vi "Main Read Data From VeriStand.vi"(8 "error in":errorcluster, 10 "Outgoing Cyclic Configuraiton":T1 {"Outgoing Cyclic Frame"."Transmit Propreties"."Transmit Time" format="%#_p"}, 11 "internal data":T6={"J1939 XNET Settings"={"XNET Database"="", "XNET Cluster"="", "CAN port"="", "Baud rate [Bd]"=0, "J1939 Network Address"=0, "Name"=0, "Termination"=0}, "j1939 queues"={"Processed Outgoing"=refnum, "Process Outgoing"=refnum, "stop notifier"=refnum, "error queue"=refnum, "active dtc"=refnum, "processed inc"=refnum}, "fgv references"={"BAM Buffer"=refnum, "CM Buffer"=refnum, "CM Gen"=refnum, "BAM Gen"=refnum, "Address Claims"=refnum, "RQST"=refnum, "scaling lut"=refnum, "data lut"=refnum, "cyclic scheduler"=refnum}, "frame in"="", "frame out"="", "timing"={"tb to j1939 queue timeout"=100, "j1939 to tb queue timeout"=100, "dtc loop period (ms)"=100, "CAN in loop period (ms)"=100, "process incoming queue timeout (ms)"=100, "Outgoing Write Decimation"=0, "process outgoing loop rate (ms)"=0, "periodic outgoing queue timeout (ms)"=10, "CAN out queue timeout (ms)"=100}}) -> ()   [LabVIEW 2013, in "J1939.lvlib"]
uses:
  J1939.lvlib
  API Types/Internal Data.ctl
  API Types/XNET Settings.ctl
  API Types/Setup Information Cluster.ctl
  API Types/CAN Outgoing Message Cluster.ctl
  API Types/Convert DTCs Cluster.ctl
  <vilib>/xnet/xnet.llb/XNET Frame CAN.ctl
  <vilib>/xnet/xnet.llb/XNET Frame Type CAN.ctl
  TP/TP List References.ctl
  BAM/BAM Buffer Connections List_Ref.ctl
  Connection Mode/Connection Mode Generation Connection Ref.ctl
  BAM/BAM Generation Connections List_Ref.ctl
  LUTs/J1939 Address Table Reference.ctl
  RQST/RQST Lookup Table Reference.ctl
  LUTs/J1939 Conversion Lookup Table Reference.ctl
  LUTs/J1939 Data Lookup Table Reference.ctl
  LUTs/Cyclic Frame Scheduler Lut Reference.ctl
  Configuration/TypeDefs/timing configuration.ctl
  CD/CD Outgoing Cyclic Configuration.ctl
  CD/CD Outgoing Cyclic Frame Pairs.ctl
  API Types/XNET Frame Event Properties.ctl
  module/configuration/Signal Mapping.ctl
  <vilib>/NI/Tag Bus/tag/Data Type.ctl
  Conversion Lookup Table Get Conversion Parameter.vi
  <vilib>/xnet/xnet.llb/XNET Convert.vi
  <vilib>/xnet/xnet.llb/XNET Convert (Signal to Frame Raw).vi
  <vilib>/NI/Tag Bus/tag/tag descriptor.lvclass
  module/configuration/J1939 configuration.lvclass
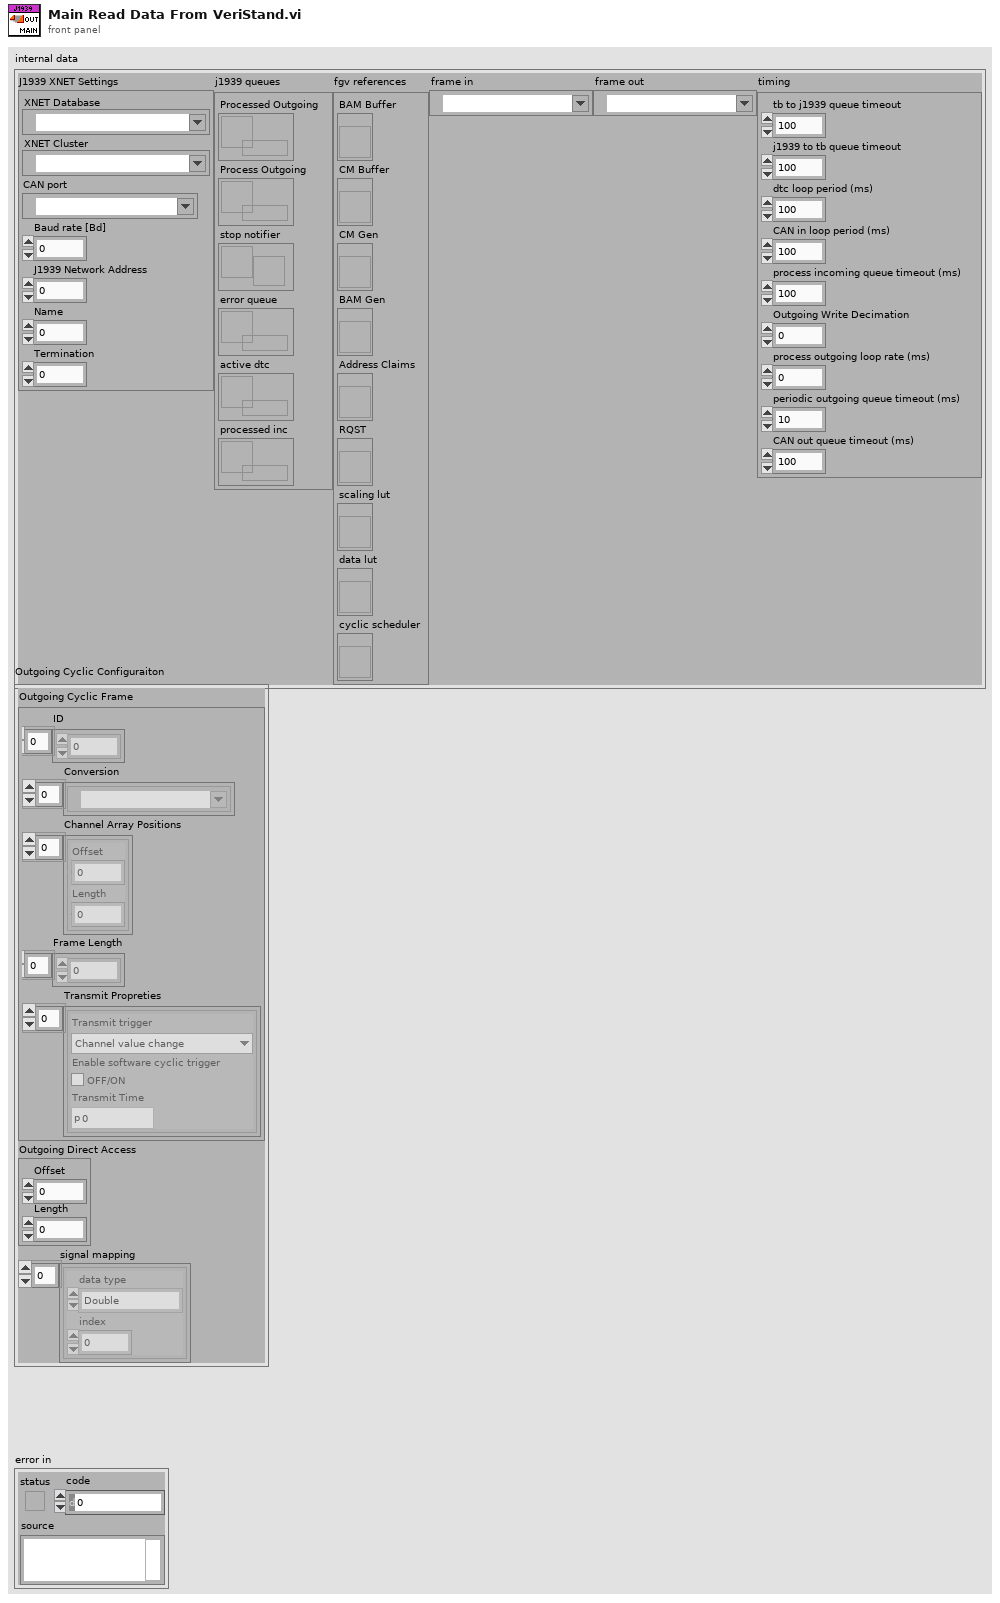
[diagram p1: front panel]
types:
  T1 = typedef "J1939.lvlib/CD Outgoing Cyclic Configuration.ctl" = cluster{"Outgoing Cyclic Frame":T2, "Outgoing Direct Access":cluster{"Offset":u32, "Length":u32}, "signal mapping":T4[]}
  T2 = typedef "J1939.lvlib/CD Outgoing Cyclic Frame Pairs.ctl" = cluster{"ID":u32[], "Conversion":refnum<k21>[], "Channel Array Positions":cluster{"Offset":u32, "Length":u32}[], "Frame Length":u32[], "Transmit Propreties":T3[]}
  T3 = typedef "J1939.lvlib/XNET Frame Event Properties.ctl" = cluster{"Transmit trigger":enum16{"Channel value change"}, "Enable software cyclic trigger":bool, "Transmit Time":dbl}
  T4 = typedef "J1939 configuration.lvclass/Signal Mapping.ctl" = cluster{"data type":T5, "index":i32}
  T5 = typedef "tag bus.lvlib/tag descriptor.lvclass/Data Type.ctl" = enum16{"Double", "Single", "I64", "I32", "I16", "I8", "U64", "U32", "U16", "U8", "Boolean", "String", "Array of Double", "Array of Single", "Array of I64", "Array of I32", "Array of I16", "Array of I8", "Array of U64", "Array of U32", "Array of U16", "Array of U8", "Array of Boolean", "Array of String"}
  T6 = typedef "J1939.lvlib/Internal Data.ctl" = cluster{"J1939 XNET Settings":T7, "j1939 queues":T8, "fgv references":T9, "frame in":refnum<k21>, "frame out":refnum<k21>, "timing":T18}
  T7 = typedef "J1939.lvlib/XNET settings.ctl" = cluster{"XNET Database":refnum<k21>, "XNET Cluster":refnum<k21>, "CAN port":refnum<k21>, "Baud rate [Bd]":u32, "J1939 Network Address":u8, "Name":u64, "Termination":u32}
  T8 = typedef "J1939.lvlib/Setup Information Cluster.ctl" = cluster{"Processed Outgoing":refnum<queue>, "Process Outgoing":refnum<queue>, "stop notifier":refnum<notifier>, "error queue":refnum<queue>, "active dtc":refnum<queue>, "processed inc":refnum<queue>}
  T9 = typedef "J1939.lvlib/TP List References.ctl" = cluster{"BAM Buffer":T10, "CM Buffer":T10, "CM Gen":T11, "BAM Gen":T12, "Address Claims":T13, "RQST":T14, "scaling lut":T15, "data lut":T16, "cyclic scheduler":T17}
  T10 = typedef "J1939.lvlib/BAM Buffer Connections List_Ref.ctl" = refnum<vi>
  T11 = typedef "J1939.lvlib/Connection Mode Generation Connection Ref.ctl" = refnum<vi>
  T12 = typedef "J1939.lvlib/BAM Generation Connections List_Ref.ctl" = refnum<vi>
  T13 = typedef "J1939.lvlib/J1939 Address Table Reference.ctl" = refnum<vi>
  T14 = typedef "J1939.lvlib/RQST Lookup Table Reference.ctl" = refnum<vi>
  T15 = typedef "J1939.lvlib/J1939 Conversion Lookup Table Reference.ctl" = refnum<vi>
  T16 = typedef "J1939.lvlib/J1939 Data Lookup Table Reference.ctl" = refnum<vi>
  T17 = typedef "J1939.lvlib/cyclic frame scheduler lut reference.ctl" = refnum<vi>
  T18 = typedef "J1939.lvlib/timing configuration.ctl" = cluster{"tb to j1939 queue timeout":i32, "j1939 to tb queue timeout":i32, "dtc loop period (ms)":i32, "CAN in loop period (ms)":i32, "process incoming queue timeout (ms)":i32, "Outgoing Write Decimation":u32, "process outgoing loop rate (ms)":i32, "periodic outgoing queue timeout (ms)":i32, "CAN out queue timeout (ms)":i32}
  T19 = typedef "J1939.lvlib/CAN Outgoing Message Cluster.ctl" = cluster{"Identifier":u32, "Data":u8[]}
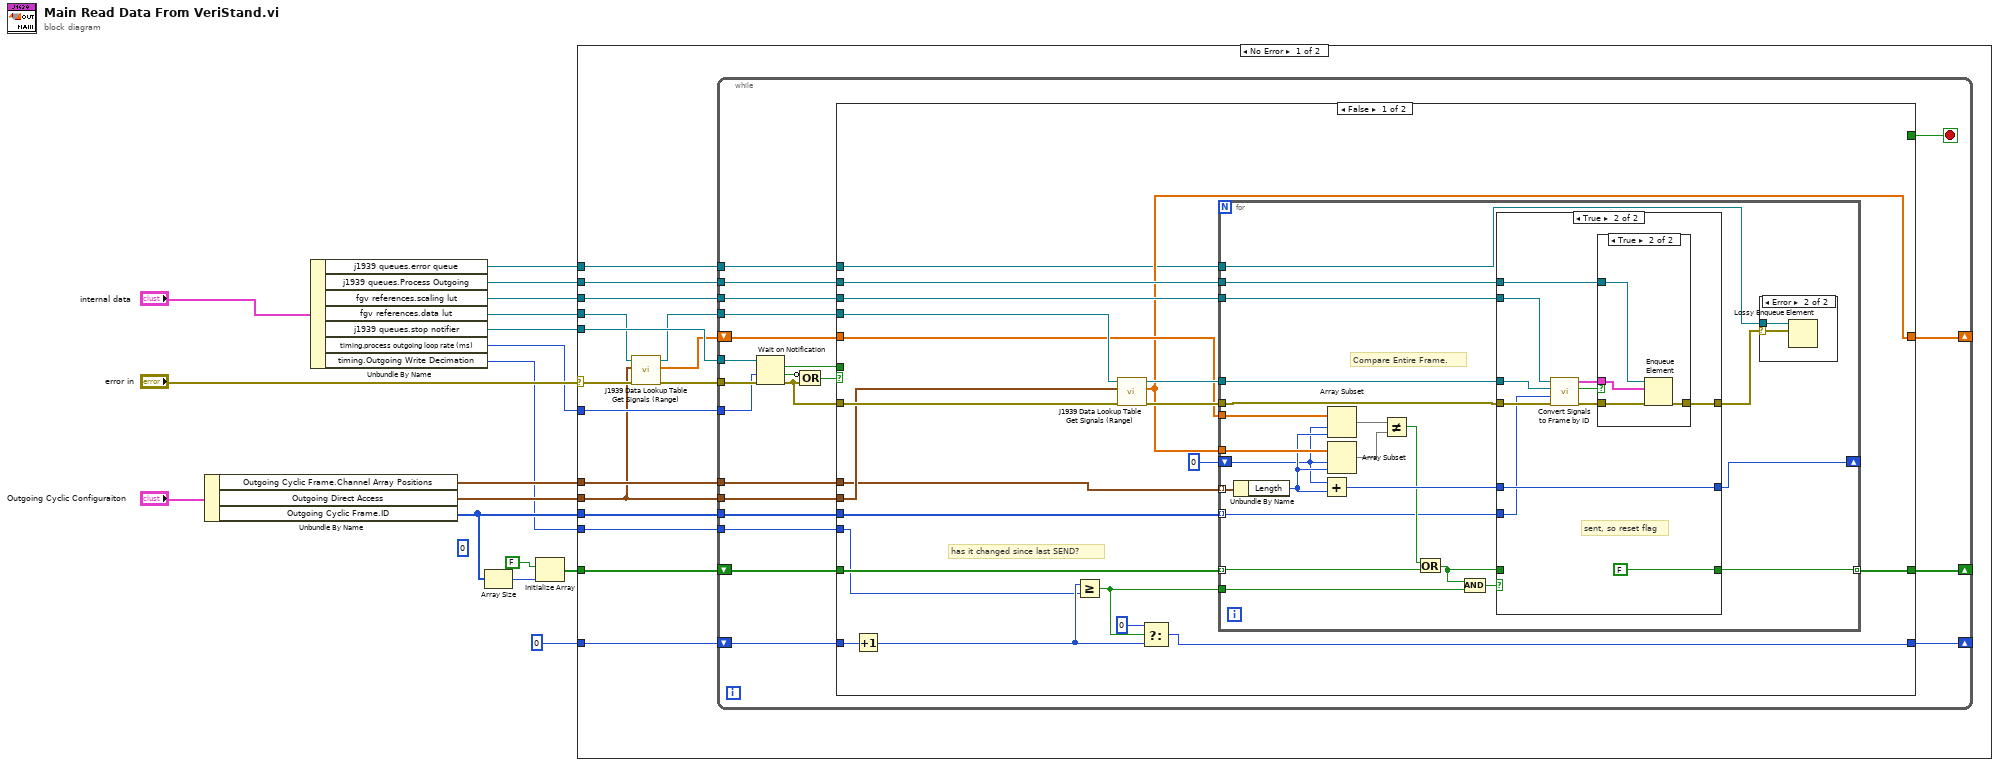
[diagram p0: block diagram]
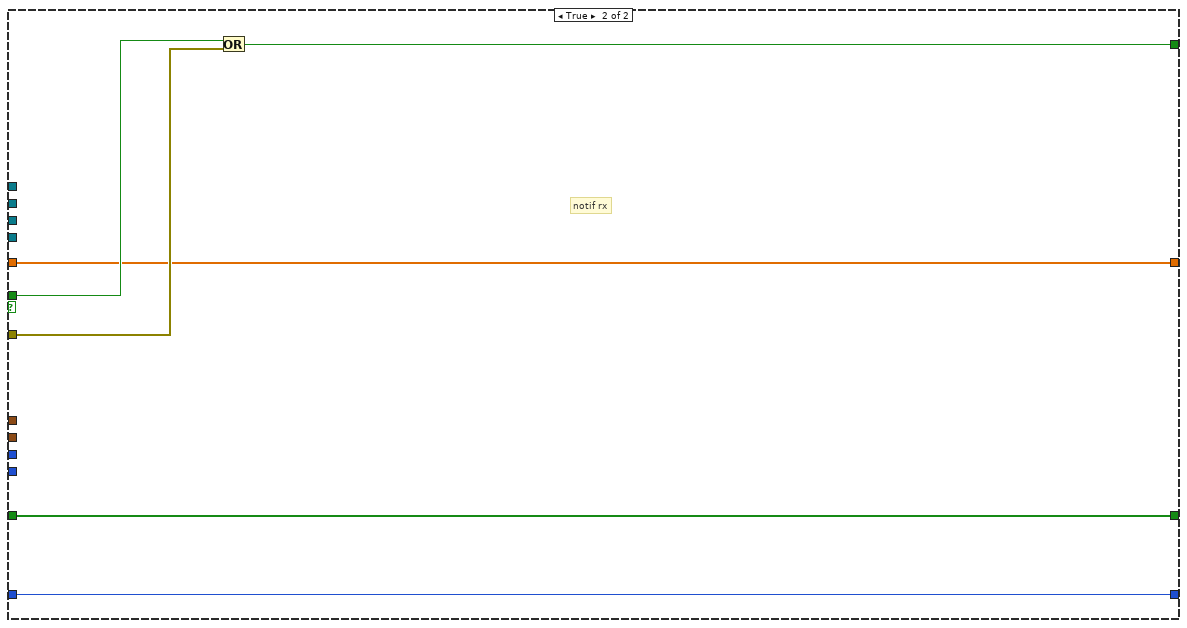
[diagram p5: hidden frame]
diagram:
  (unwired) u32 0 ("Write Decimation")
  n1 = Unbundle By Name("Outgoing Cyclic Configuraiton") -> ("Outgoing Cyclic Frame.Channel Array Positions"=w6:cluster{"Offset":u32, "Length":u32}[], "Outgoing Direct Access"=w7:cluster{"Offset":u32, "Length":u32}, "Outgoing Cyclic Frame.ID"=w11:u32[])
  n2 = Unbundle By Name("internal data") -> ("j1939 queues.error queue"=w3:refnum<queue>, "j1939 queues.Process Outgoing"=w4:refnum<queue>, "fgv references.scaling lut"=w5:T15, "fgv references.data lut"=w8:T16, "j1939 queues.stop notifier"=w16:refnum<notifier>, "timing.process outgoing loop rate (ms)"=w1:i32, "timing.Outgoing Write Decimation"=w2:u32)
  n3 = Array Size(array=w11) -> (size(s)=w13:i32)
  n4 = Initialize Array(FALSE, w13) -> (w10:bool[])
  n5 = case shown="No Error" "error in" {
    selector: "error in" -> [w24 _]
    tunnel: w16 -> [w33 _]
    tunnel: w2 -> [w32 _]
    tunnel: w11 -> [w31 _]
    tunnel: w10 -> [w30 _]
    tunnel: u32 0 -> [w29 _]
    tunnel: w8 -> [w20 _]
    tunnel: w7 -> [w21 _]
    tunnel: w6 -> [w28 _]
    tunnel: w5 -> [w27 _]
    tunnel: w4 -> [w26 _]
    tunnel: w1 -> [w25 _]
    tunnel: w3 -> [w18 _]
    frame No Error {
      n6 = call "J1939 Data Lookup Table Get Signals (Range).vi"("error in (no error)"=w24, "Direct Access"=w21, "Ref in"=w20) -> ("error out"=w23:errorcluster, "Signals"=w22:dbl[], "vi reference"=w19:T16)  [unwired: 6 in]
      n7 = while {
        tunnel: w33 -> [w54]
        tunnel: w23 -> [w55]
        tunnel: w32 -> [w48]
        tunnel: w31 -> [w47]
        shift-right: [w46] -> _
        shift-left: w30 -> [w45]
        shift-right: [w43] -> _
        shift-left: w29 -> [w44]
        tunnel: w19 -> [w42]
        tunnel: w21 -> [w41]
        tunnel: w28 -> [w40]
        tunnel: w27 -> [w39]
        tunnel: w26 -> [w38]
        shift-right: [w36] -> _
        shift-left: w22 -> [w37]
        tunnel: w25 -> [w35]
        tunnel: w18 -> [w34]
        stop <- w49 stop-if-true
        n8 = Wait on Notification(notifier=w54, timeout in ms (-1)=w35, error in (no error)=w55) -> (notification=w50:bool, timed out?=w53:bool, error out=w51:errorcluster)  [unwired: 1 in, 1 out]
        n9 = Compound Arithmetic op=OR(invert w53, w51) -> (w52:bool)
        n10 = case shown="False" w52 {
          tunnel: w51 -> [w71 w123]
          tunnel: w50 -> [_ w125]
          tunnel: [_ w124] -> w49
          tunnel: w48 -> [w70 _]
          tunnel: w47 -> [w66 _]
          tunnel: [w74 w122] -> w46
          tunnel: w45 -> [w75 w122]
          tunnel: w44 -> [w76 w121]
          tunnel: [w72 w121] -> w43
          tunnel: w42 -> [w69 _]
          tunnel: w41 -> [w68 _]
          tunnel: w40 -> [w67 _]
          tunnel: w39 -> [w65 _]
          tunnel: w38 -> [w64 _]
          tunnel: w37 -> [w58 w120]
          tunnel: [w57 w120] -> w36
          tunnel: w34 -> [w56 _]
          frame False {
            # "has it changed since last SEND?"
            n11 = Increment(x=w76) -> (x+1=w73:u32)
            n12 = Greater Or Equal?(x=w73, y=w70) -> (x >= y?=w60:bool)
            n13 = call "J1939 Data Lookup Table Get Signals (Range).vi"("error in (no error)"=w71, "Direct Access"=w68, "Ref in"=w69) -> ("error out"=w63:errorcluster, "Signals"=w57:dbl[], "vi reference"=w62:T16)  [unwired: 6 in]
            n14 = Select(t=0, s=w60, f=w73) -> (s? t:f=w72:u32)
            n15 = for {
              tunnel: w67 -> [w98] mode=indexing
              tunnel: w62 -> [w91]
              tunnel: w58 -> [w97]
              tunnel: w57 -> [w96]
              shift-right: [w85] -> _
              shift-left: u32 0 -> [w94]
              tunnel: w64 -> [w92]
              tunnel: w65 -> [w90]
              tunnel: [w89] -> w74 mode=indexing
              tunnel: w75 -> [w84] mode=indexing
              tunnel: w60 -> [w87]
              tunnel: w66 -> [w79] mode=indexing
              tunnel: w63 -> [w93]
              tunnel: w56 -> [w77]
              # "Compare Entire Frame."
              n16 = Unbundle By Name(w98) -> ("Length"=w95:u32)
              n17 = Add(x=w94, y=w95) -> (x+y=w86:u32)
              n18 = Array Subset(array=w97, index=w94, length=w95) -> (w80:dbl[])
              n19 = Array Subset(array=w96, index=w94, length=w95) -> (w81:dbl[])
              n20 = Not Equal?(x=w80, y=w81) -> (x != y?=w83:bool)
              n21 = Or(x=w83, y=w84) -> (x .or. y?=w82:bool)
              n22 = Compound Arithmetic op=AND(w82, w87) -> (w88:bool)
              n23 = case shown="True" w88 {
                tunnel: w93 -> [w103 w112]
                tunnel: [w103 w114] -> w78
                tunnel: w92 -> [_ w113]
                tunnel: w79 -> [_ w105]
                tunnel: w91 -> [_ w109]
                tunnel: w90 -> [_ w108]
                tunnel: [w101 FALSE] -> w89
                tunnel: w86 -> [w102 w106]
                tunnel: [w102 w106] -> w85
                tunnel: w82 -> [w101 _]
                frame False {
                }
                frame True {
                  # "sent, so reset flag"
                  n24 = call "Convert Signals to Frame by ID.vi"("error in (no error)"=w112, "ID"=w105, "Data Ref"=w109, "Conv Ref"=w108) -> ("error out"=w111:errorcluster, "Found?"=w104:bool, "Frame"=w110:T19)  [unwired: 5 in]
                  n25 = case shown="True" w104 {
                    tunnel: [w115 w119] -> w114
                    tunnel: w113 -> [_ w118]
                    tunnel: w111 -> [w115 w117]
                    tunnel: w110 -> [_ w116]
                    frame False {
                    }
                    frame True {
                      n26 = Enqueue Element(queue=w118, element=w116, error in (no error)=w117) -> (error out=w119:errorcluster)  [unwired: 3 out]
                    }
                  }
                }
              }
              n27 = case shown="Error" w78 {
                selector: w78 -> [_ w99]
                tunnel: w77 -> [_ w100]
                frame No Error {
                }
                frame Error {
                  n28 = Lossy Enqueue Element(queue=w100, element=w99) -> ()  [unwired: 1 in, 4 out]
                }
              }
            }
          }
          frame True {
            # "notif rx"
            n29 = Or(x=w125, y=w123) -> (x .or. y?=w124:bool)
          }
        }
      }
    }
    frame Error {
    }
  }
